vi "ALLPROPS1dll.vi"(8 "error in (no error)":errorcluster, 11 "Inputs":T1) -> (0 "error out":errorcluster, 3 "Outputs":T2)   [LabVIEW 2016]
doc: "subroutine ALLPROP1dll(hOut, iUnits, T, D, z, c, ierr, herr, hOut_length, herr_length)\n\nShort version of subroutine ALLPROPS that eliminates the arrays but allows the calculation of only one property\nat a time. All inputs and outputs are described in the ALLPROPS routine.\n\nINPUTS:\nhOut -- Input string of properties to calculate (of any length). Inputs can be separated by spaces, commas, semicolons, or bars, but should not be mixed. For example, a proper string would be hOut=’T,P,D,H,E,S’, whereas an improperly defined string would be hOut=’T,P;D H|E,S’. Use of lower or upper case is not important. Some properties will return multiple values, for example, hOut=’F,Fc,XMOLE’ will return 12 properties for a four component system, these being F(1), F(2), F(3), F(4), Fc(1), Fc(2), etc. To retrieve the property of a single component, use, for example, hOut=’XMOLE(2),XMOLE(3)’\niUnits -- See subroutine REFPROP for a complete description of the iUnits input\nvalue. A negative value for iUnits indicates that the input temperature is given in K and\ndensity in mol/dm^3, (Refprop default units), otherwise T and D will be converted first to K\nand mol/dm^3. Do not use the negative value for the iUnits parameter everywhere, only in\nthis one situation.\nT --Temperature, with units based on the value of iUnits.\nD -- Density, with units based on the value of iUnits.\nz -- Composition on a mole or mass basis (array of size ncmax=20)\n\nOUTPUTS:\nc -- Output value (array of size 200 dimensioned as double precision) The number -9999970 will be returned when errors occur or no input was requested.\nierr -- Error flag\nherr -- Error string (character*255)\nhOut_length -- length of variable hOut (default: 255)\nherr_length -- length of variable herr (default: 255)"
uses:
  REFPROP.DLL
panel:
  # "REFPROP-ALLPROP1dll.vi"
  # "void  ALLPROP1dll(CStr hOut, int32_t *iUnits, double *T, double *D, double *z, double *c, int32_t *ierr, CStr herr, int32_t *hOut_Length, int32_t *herr_length);"
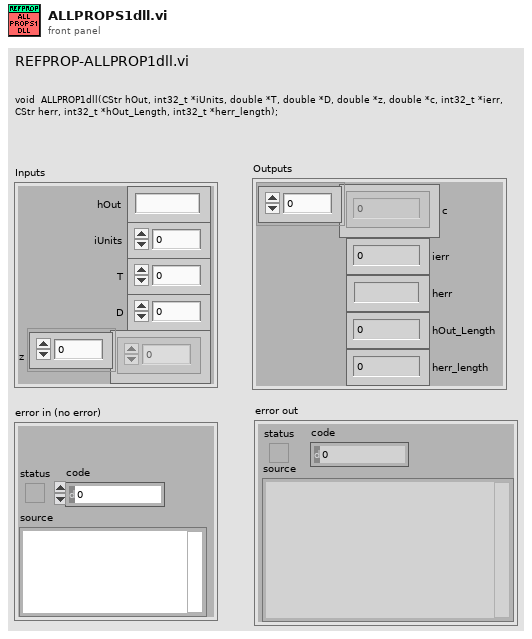
[diagram p1: front panel]
types:
  T1 = cluster{"hOut":string, "iUnits":i32, "T":dbl, "D":dbl, "z":dbl[]}
  T2 = cluster{"c":dbl[], "ierr":i32, "herr":string, "hOut_Length":i32, "herr_length":i32}
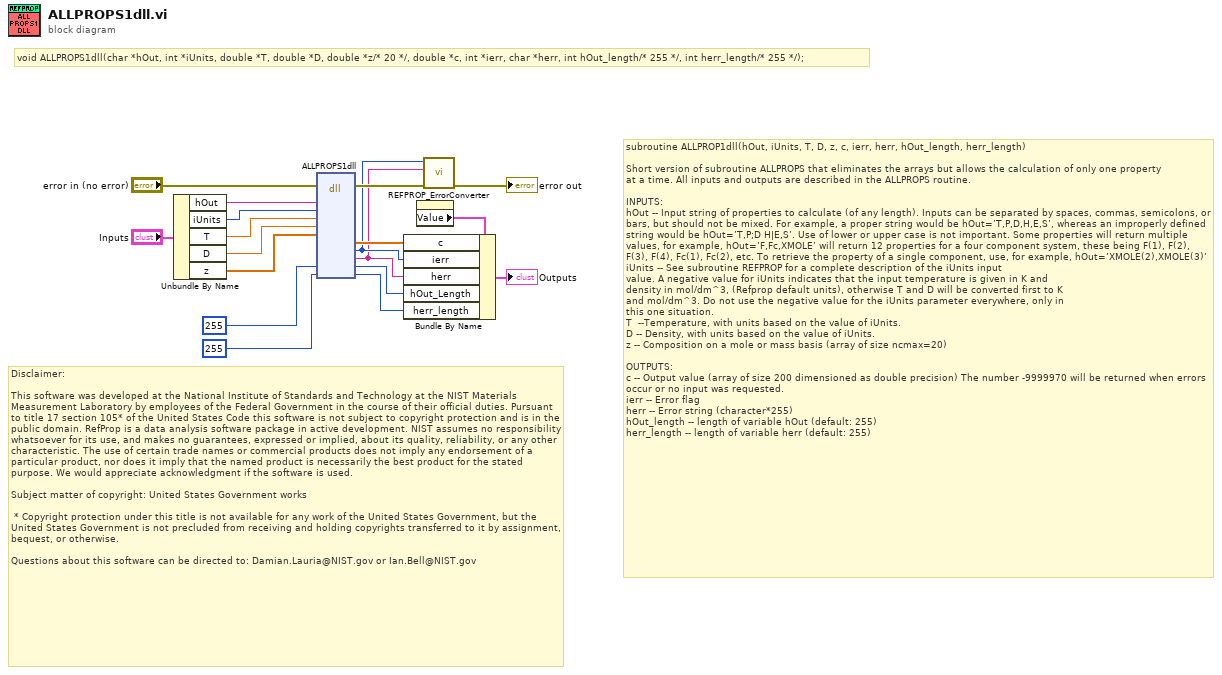
[diagram p0: block diagram]
diagram:
  # "void ALLPROPS1dll(char *hOut, int *iUnits, double *T, double *D, double *z/* 20 */, double *c, int *ierr, char *herr, int hOut_length/* 255 */, int herr_length/* 255 */);"
  # "subroutine ALLPROP1dll(hOut, iUnits, T, D, z, c, ierr, herr, hOut_length, herr_length)\n\nShort version of subroutine ALLPROPS that eliminates the arrays but allows the calculation of only one property\nat a time. All inputs and outputs are described in the ALLPROPS routine.\n\nINPUTS:\nhOut -- Input string of properties to calculate (of any length). Inputs can be separated by spaces, commas, semicolons, or bars, but should not be mixed. For example, a proper string would be hOut=’T,P,D,H,E,S’, whereas an improperly defined string would be hOut=’T,P;D H|E,S’. Use of lower or upper case is not important. Some properties will return multiple values, for example, hOut=’F,Fc,XMOLE’ will return 12 properties for a four component system, these being F(1), F(2), F(3), F(4), Fc(1), Fc(2), etc. To retrieve the property of a single component, use, for example, hOut=’XMOLE(2),XMOLE(3)’\niUnits -- See subroutine REFPROP for a complete description of the iUnits input\nvalue. A negative value for iUnits indicates that the input temperature is given in K and\ndensity in mol/dm^3, (Refprop default units), otherwise T and D will be converted first to K\nand mol/dm^3. Do not use the negative value for the iUnits parameter everywhere, only in\nthis one situation.\nT  --Temperature, with units based on the value of iUnits.\nD -- Density, with units based on the value of iUnits.\nz -- Composition on a mole or mass basis (array of size ncmax=20)\n\nOUTPUTS:\nc -- Output value (array of size 200 dimensioned as double precision) The number -9999970 will be returned when errors occur or no input was requested.\nierr -- Error flag\nherr -- Error string (character*255)\nhOut_length -- length of variable hOut (default: 255)\nherr_length -- length of variable herr (default: 255)"
  # "Disclaimer:\n\nThis software was developed at the National Institute of Standards and Technology at the NIST Materials Measurement Laboratory by employees of the Federal Government in the course of their official duties. Pursuant to title 17 section 105* of the United States Code this software is not subject to copyright protection and is in the public domain. RefProp is a data analysis software package in active development. NIST assumes no responsibility whatsoever for its use, and makes no guarantees, expressed or implied, about its quality, reliability, or any other characteristic. The use of certain trade names or commercial products does not imply any endorsement of a particular product, nor does it imply that the named product is necessarily the best product for the stated purpose. We would appreciate acknowledgment if the software is used.\n \nSubject matter of copyright: United States Government works\n  \n * Copyright protection under this title is not available for any work of the United States Government, but the United States Government is not precluded from receiving and holding copyrights transferred to it by assignment, bequest, or otherwise.\n\nQuestions about this software can be directed to: Damian.Lauria@NIST.gov or Ian.Bell@NIST.gov"
  n1 = Unbundle By Name("Inputs") -> ("hOut"=w6:string, "iUnits"=w5:i32, "T"=w4:dbl, "D"=w3:dbl, "z"=w2:dbl[])
  n2 = dll-call lib="S:/009 - Testing/02 - Performance Testing/REFPROP/refprop.*" fn="ALLPROPS1dll"(error in="error in (no error)", "hOut"=w6, "iUnits"=w5, "T"=w4, "D"=w3, "z"=w2, "hOut_Length"=255 ("ln"), "herr_length"=255 ("ln")) -> (error out=w16:errorcluster, "c"=w12:dbl[], "ierr"=w11:i32, "herr"=w10:string, "hOut_Length"=w9:i32, "herr_length"=w8:i32)  [unwired: 11 in, 1 out]
  n3 = property on="Outputs" class="Clust (strict)"() -> ("Value"=w14:T2)  [unwired: 2 in, 2 out]
  n4 = Bundle By Name(cluster=w14, "c"=w12, "ierr"=w11, "herr"=w10, "hOut_Length"=w9, "herr_length"=w8) -> (→"Outputs":T2)
  n5 = call "REFPROP_ErrorConverter.vi"("error in (no error)"=w16, "Error Message"=w10, "Error Code"=w11) -> ("error out"=→"error out":errorcluster)  [unwired: 8 in]
